vi "Connect Multi Frame.vi"(8 "error in (no error)":errorcluster, 11 "BML Frame Array":refnum<class "BML_Frame_Root.lvclass">[](array[class])) -> (0 "error out":errorcluster, 3 "Connected Frame Contents":string)   [LabVIEW 2016, in "BML_DigiPattern_Generator.lvclass"]
uses:
  BML_DigiPattern_Generator.lvclass
  BML_Frame_Root/BML_Frame_Root.lvclass
  BML_Frame_Root/BML_Frame_Root.lvclass/BML_Frame_Root.ctl
  BML_Frame_Root/Special Frame.ctl
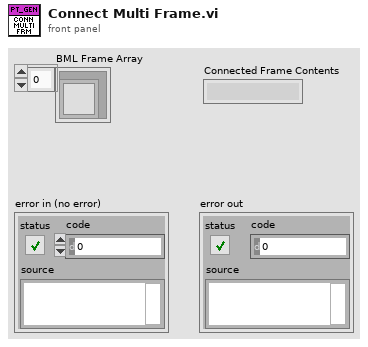
[diagram p1: front panel]
types:
  T1 = typedef "BML_Frame_Root.lvclass/Special Frame.ctl" = enum16{"Sync Header", "Protocol Header", "SW Trig", "SetID State", "Out SetID State", "SW Reset", "Wait"}
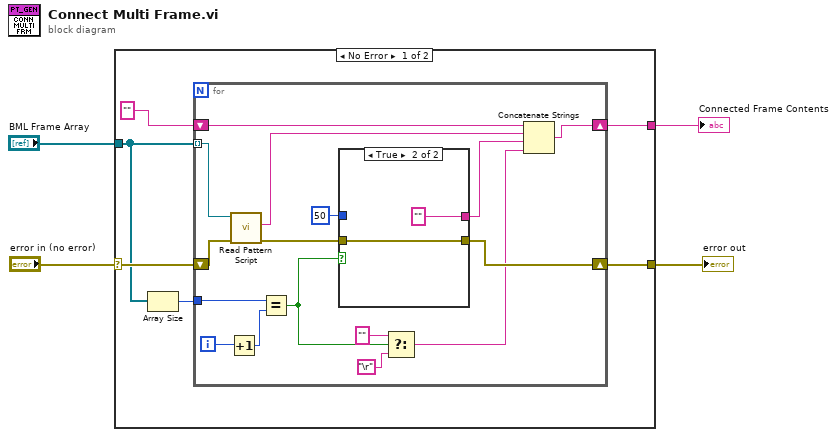
[diagram p0: block diagram]
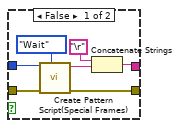
[diagram p2: hidden frame]
diagram:
  n1 = case shown="No Error" "error in (no error)" {
    selector: "error in (no error)" -> [w8 w36]
    tunnel: "BML Frame Array" -> [w7 _]
    tunnel: [w9 w36] -> w3
    tunnel: [w5 _] -> w1
    frame No Error {
      n2 = Array Size(array=w7) -> (size(s)=w6:i32)
      n3 = for {
        tunnel: w7 -> [w26] mode=indexing
        shift-right: [w16] -> w9
        shift-left: w8 -> [w25]
        shift-right: [w24] -> w5
        shift-left: "" -> [w23]
        tunnel: w6 -> [w15]
        i -> [w22]
        n4 = Increment(x=w22) -> (x+1=w21:i32)
        n5 = call "Read Pattern Script.vi"("error in (no error)"=w25, "BML_Frame_Root in"=w26) -> ("error out"=w17:errorcluster, "Pattern Script"=w14:string)  [unwired: 7 in, 1 out]
        n6 = Equal?(x=w15, y=w21) -> (x = y?=w18:bool)
        n7 = case shown="True" w18 {
          tunnel: w17 -> [w33 w34]
          tunnel: [w32 w34] -> w16
          tunnel: u32 50 ("Num of Timeset") -> [w31 _]
          tunnel: [w28 "" ("string out")] -> w11
          frame False {
            n8 = call "Create Pattern Script(Special Frames).vi"("Special Frame Type"=Special_Frame."Wait", "error in (no error)"=w33, "Num of Timeset"=w31) -> ("error out"=w32:errorcluster, "string out"=w29:string)  [unwired: 7 in]
            n9 = Concatenate Strings("\r", w29) -> (w28:string)
          }
          frame True {
          }
        }
        n10 = Select(t="", s=w18, f="\r") -> (s? t:f=w12:string)
        n11 = Concatenate Strings(w23, w14, w11, w12) -> (w24:string)
      }
    }
    frame Error {
    }
  }
  "error out" <- w3
  "Connected Frame Contents" <- w1
